vi "UpdateLogFile.vi"(6 "Data":string[](array[string]), 7 "Log?":bool, 8 "ErrorIn":errorcluster, 11 "LogFile":path) -> (0 "ErrorOut":errorcluster)   [LabVIEW 2018]
doc: "This VI provides simple sample code for logging an array of strings (could be converted numerics) with a date and time stamp to a file specified as one of the inputs to the VI.s\n\nCopyright © 2011 Epimedia, Inc. All Rights Reserved.\n\nThe Epimedia Application Library is Copyright © 2009-2011 Epimedia, Inc. \nAll Rights Reserved. Used under license."
panel:
  # "Copyright © 2011 Epimedia, Inc. All Rights Reserved.\n\nThe Epimedia Application Library is Copyright © 2009-2011 Epimedia, Inc. \nAll Rights Reserved. Used under license."
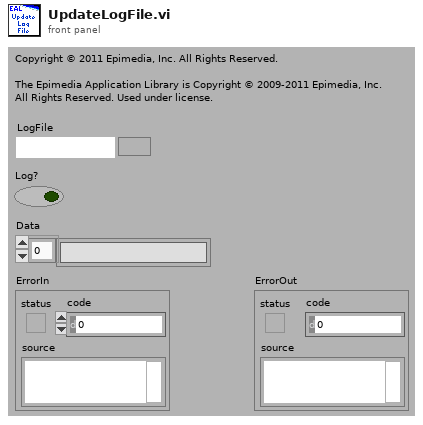
[diagram p1: front panel]
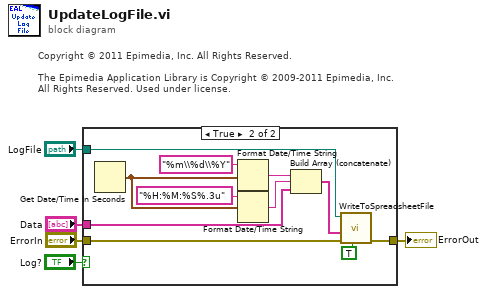
[diagram p0: block diagram]
diagram:
  # "Copyright © 2011 Epimedia, Inc. All Rights Reserved.\n\nThe Epimedia Application Library is Copyright © 2009-2011 Epimedia, Inc. \nAll Rights Reserved. Used under license."
  n1 = case shown="True" "Log?" {
    tunnel: "ErrorIn" -> [w6 w11]
    tunnel: [w6 w10] -> w2
    tunnel: "Data" -> [_ w12]
    tunnel: "LogFile" -> [_ w8]
    frame False {
    }
    frame True {
      n2 = Get Date/Time In Seconds() -> (seconds since 1Jan1904=w16:timestamp)
      n3 = Format Date/Time String(time format string (%c)="%m\\%d\\%Y", seconds (now)=w16) -> (date/time string=w14:string)  [unwired: 1 out]
      n4 = Format Date/Time String(time format string (%c)="%H:%M:%S%.3u", seconds (now)=w16) -> (date/time string=w13:string)  [unwired: 1 out]
      n5 = Build Array (concatenate)(w14, w13, w12) -> (w9:string[])
      n6 = call "WriteToSpreadsheetFile.vi"("Append?(NewFile:F)"=TRUE ("append to file? (new file:F)"), "ErrorIn"=w11, "1D-Data"=w9, "FilePath(DialogIfEmpty)"=w8) -> ("ErrorOut"=w10:errorcluster)  [unwired: 4 in, 3 out]
    }
  }
  "ErrorOut" <- w2
